vi "NF WF1973_74 CHAN Copy.vi"(8 "error in (no error)":errorcluster caption="Error IN", 10 "Copy(Ch1>Ch2)":bool, 11 "VISAsession":refnum<visa-resource-name>) -> (0 "error out":errorcluster caption="Error OUT", 3 "CopyVISAsession":refnum<visa-resource-name>)   [LabVIEW 2010]
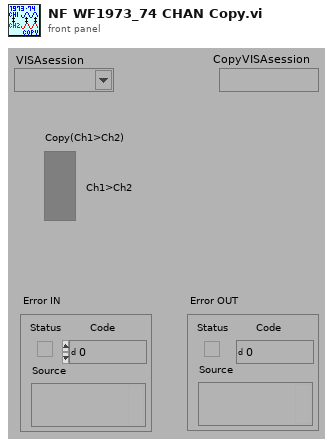
[diagram p1: front panel]
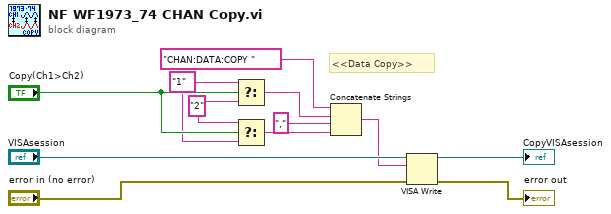
[diagram p0: block diagram]
diagram:
  w1 = "1"
  w2 = "2"
  # "<<Data Copy>>"
  n1 = Select(t=w1, s="Copy(Ch1>Ch2)", f=w2) -> (s? t:f=w6:string)
  n2 = Select(t=w2, s="Copy(Ch1>Ch2)", f=w1) -> (s? t:f=w5:string)
  n3 = Concatenate Strings("CHAN:DATA:COPY " ("文字列"), w6, ",", w5) -> (w8:string)
  n4 = VISA Write(VISA resource name="VISAsession", write buffer=w8, error in (no error)="error in (no error)") -> (VISA resource name out=→"CopyVISAsession":refnum<visa-resource-name>, error out=→"error out":errorcluster)  [unwired: 1 out]
